vi "Open VISA by COM Descriptor.vi"(8 "error in (no error)":errorcluster, 11 "COM descriptor":string) -> (0 "error out":errorcluster, 3 "VISA resource name out":refnum<visa-resource-name>)   [LabVIEW 2020, in "Get COM Descriptor.lvlib"]
doc: "Open VISA by COM port descriptor. Generates error if multiple COM ports match given descriptor."
uses:
  Get COM Descriptor.lvlib
  <vilib>/Utility/error.llb/Error Cluster From Error Code.vi
  <vilib>/ErrorRing/Error Ring.xnode
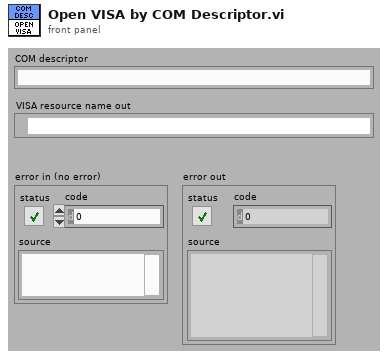
[diagram p1: front panel]
types:
  T1 = typedef "Get COM Descriptor.lvlib/COM port.ctl" = cluster{"port":string, "descriptor":string}
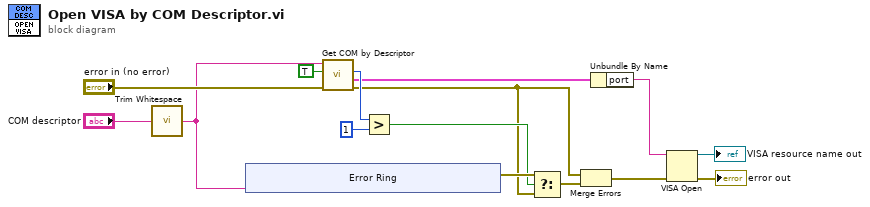
[diagram p0: block diagram]
diagram:
  n1 = call <vilib>:"Trim Whitespace.vi"("string"="COM descriptor") -> ("trimmed string"=w11:string)  [unwired: 1 in]
  n2 = xnode "Error Ring"("parameter 0"=w11) -> ("error out"=w14:errorcluster)
  n3 = call "Get COM by Descriptor.vi"("error in (no error)"="error in (no error)", "Generate error if no COM port found? (False)"=TRUE, "COM descriptor"=w11) -> ("error out"=w6:errorcluster, "First COM port"=w4:T1, "COM ports count"=w9:i32)  [unwired: 5 in, 1 out]
  n4 = Greater?(x=w9, y=1) -> (0:w7:bool)
  n5 = Select(t=w14, s=w7, f=w6) -> (s? t:f=w13:errorcluster)
  n6 = Merge Errors(w6, w13) -> (w5:errorcluster)
  n7 = Unbundle By Name(w4) -> ("port"=w3:string)
  n8 = VISA Open(error in (no error)=w5, VISA resource name=w3) -> (VISA resource name=→"VISA resource name out":refnum<visa-resource-name>, error out=→"error out":errorcluster)  [unwired: 3 in]
